vi "Set Domain.vi"(7 "target Domain":refnum<class "NI_Domain.lvclass">, 8 "error in (no error)":errorcluster, 10 "domain":variant, 11 "PDE in":refnum<class "NI_PDE.lvclass">) -> (0 "error out":errorcluster, 3 "PDE out":refnum<class "NI_PDE.lvclass">)   [LabVIEW 2020, in "NI_PDE.lvlib" / "NI_PDE.lvclass"]
uses:
  <vilib>/gmath/pde.llb/PDEClass/NI_PDE.lvclass
  <vilib>/gmath/pde.llb/DomainClass/NI_Domain.lvclass
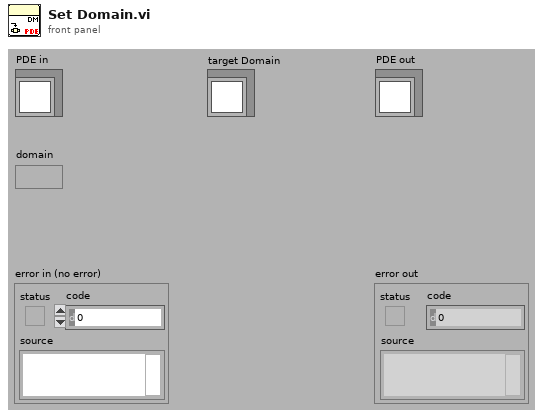
[diagram p1: front panel]
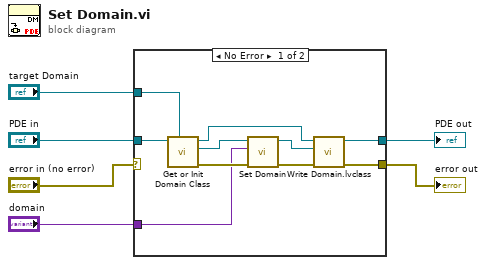
[diagram p0: block diagram]
diagram:
  n1 = case shown="No Error" "error in (no error)" {
    selector: "error in (no error)" -> [_ w18]
    tunnel: "PDE in" -> [w16 w17]
    tunnel: [w14 w17] -> w6
    tunnel: [w13 w18] -> w5
    tunnel: "target Domain" -> [w7 _]
    tunnel: "domain" -> [w8 _]
    frame No Error {
      n2 = call <vilib>:"Get or Init Domain Class.vi"("target Domain"=w7, "PDE out"=w16) -> ("error out"=w12:errorcluster, "Domain out"=w11:refnum<class "NI_Domain.lvclass">, "PDE in"=w15:refnum<class "NI_PDE.lvclass">)  [unwired: 1 in, 6 out]
      n3 = call-dynamic "Set Domain.vi"("error in (no error)"=w12, "domain"=w8, "Domain in"=w11) -> ("error out"=w9:errorcluster, "Domain out"=w10:refnum<class "NI_Domain.lvclass">)  [unwired: 7 out]
      n4 = call-dynamic "Write Domain.lvclass.vi"("error in (no error)"=w9, "Domain.lvclass"=w10, "PDE.lvclass in"=w15) -> ("error out"=w13:errorcluster, "PDE.lvclass out"=w14:refnum<class "NI_PDE.lvclass">)  [unwired: 7 out]
    }
    frame Error {
    }
  }
  "PDE out" <- w6
  "error out" <- w5
